vi "ReadDiscreteInputs.vi"(8 "error in":errorcluster, 11 "Modbus instance in":refnum<class "Modbus API.lvclass">) -> (0 "error out":errorcluster, 2 "discrete inputs":bool[](array[boolean]), 3 "Modbus instance out":refnum<class "Modbus API.lvclass">)   [LabVIEW 2016]
uses:
  <vilib>/NI/Modbus Library/API/Modbus API.lvclass
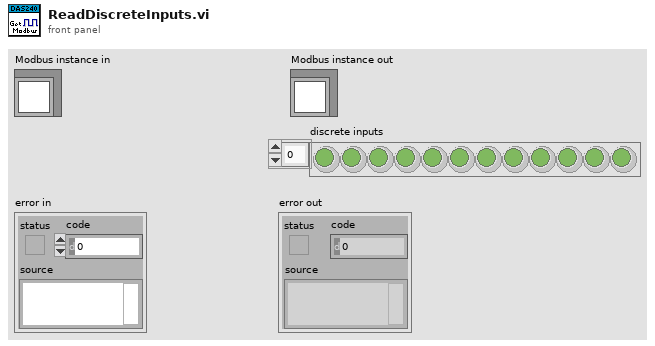
[diagram p1: front panel]
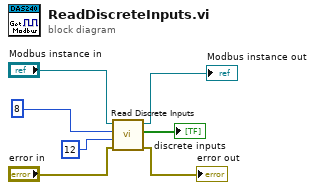
[diagram p0: block diagram]
diagram:
  n1 = call-dynamic "Read Discrete Inputs.vi"("error in"="error in", "number of inputs"=u16 12, "starting address"=u16 8, "Modbus instance in"="Modbus instance in") -> ("error out"=→"error out":errorcluster, "discrete inputs"=→"discrete inputs":bool[], "Modbus instance out"=→"Modbus instance out":refnum<class "Modbus API.lvclass">)  [unwired: 5 in]
